vi "Adjust ROI.vi"(10 "Horizontal Pixel ROI IN":cluster{i64, i64}) -> (2 "Horizontal Pixel ROI OUT":cluster{i64, i64})   [LabVIEW 2020]
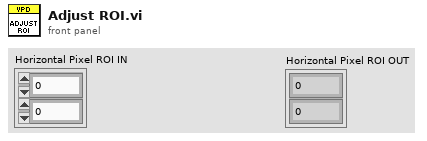
[diagram p1: front panel]
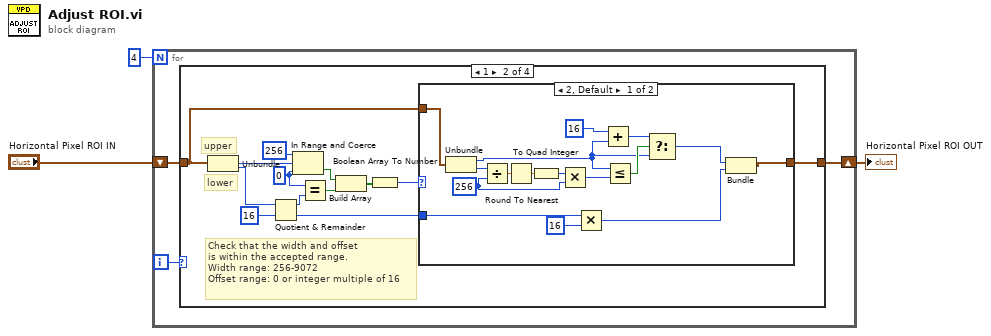
[diagram p0: block diagram]
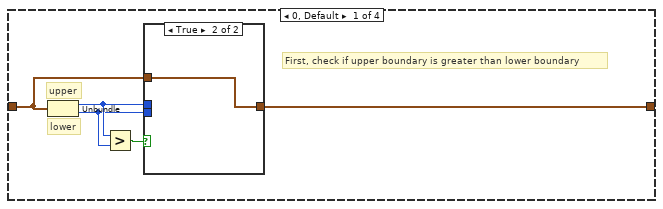
[diagram p2: hidden frame]
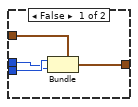
[diagram p3: hidden frame]
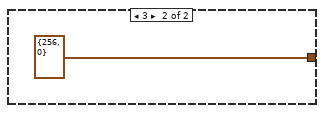
[diagram p4: hidden frame]
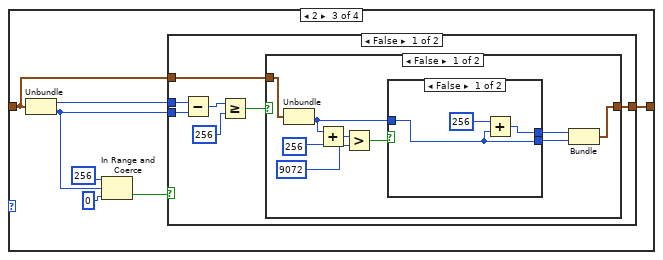
[diagram p5: hidden frame]
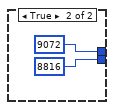
[diagram p6: hidden frame]
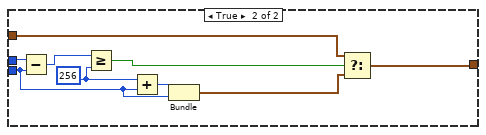
[diagram p8: hidden frame]
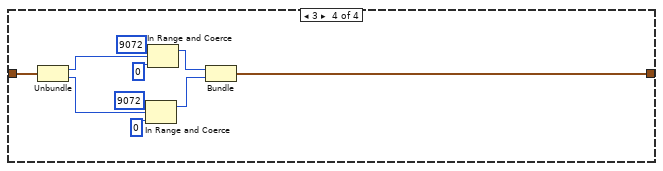
[diagram p9: hidden frame]
diagram:
  n1 = for {
    N: 4 -> [_]
    shift-right: [w5] -> w2
    shift-left: "Horizontal Pixel ROI IN" -> [w6]
    i -> [w4]
    n2 = case shown="1" w4 {
      tunnel: w6 -> [w10 w24 w48 w94]
      tunnel: [w7 w23 w47 w87] -> w5
      frame 0, Default {
        # "First, check if upper boundary is greater than lower boundary"
        # "lower"
        # "upper"
        n3 = Unbundle(w10) -> (w9:i64, w8:i64)
        n4 = Greater?(x=w9, y=w8) -> (0:w11:bool)
        n5 = case shown="True" w11 {
          tunnel: w10 -> [w15 w16]
          tunnel: w9 -> [w12 _]
          tunnel: w8 -> [w14 _]
          tunnel: [w13 w16] -> w7
          frame False {
            n6 = Bundle(cluster=w15, w14, w12) -> (w13:cluster{i64, i64})
          }
          frame True {
          }
        }
      }
      frame 1 {
        w19 = i64 0 ("lower limit")
        # "Check that the width and offset\nis within the accepted range.\nWidth range: 256-9072\nOffset range: 0 or integer multiple of 16"
        # "upper"
        # "lower"
        n7 = Unbundle(w24) -> (w29:i64, w22:i64)
        n8 = Quotient & Remainder(x=w22, y=i64 16) -> (x-y*floor(x/y)=w20:i64, floor(x/y)=w17:i64)
        n9 = In Range and Coerce(upper limit=i64 256, x=w29, lower limit=w19) -> (In Range?=w27:bool)  [unwired: 1 out]
        n10 = Equal?(x=w19, y=w20) -> (x = y?=w18:bool)
        n11 = Build Array(w27, w18) -> (w26:bool[])
        n12 = Boolean Array To Number(Boolean array=w26) -> (number=w25:u8)
        n13 = case shown="2, Default" w25 {
          tunnel: w24 -> [w33 _]
          tunnel: [w34 cluster{i64, i64} {256, 0} ("Horizontal Pixel slider")] -> w23
          tunnel: w17 -> [w32 _]
          frame 2, Default {
            w41 = i64 256 ("y")
            n14 = Unbundle(w33) -> (w38:i64, w45:i64)
            n15 = Divide(x=w45, y=w41) -> (x/y=w44:dbl)
            n16 = Round To Nearest(number=w44) -> (nearest integer value=w43:dbl)
            n17 = To Quad Integer(1:w43) -> (0:w42:i64)
            n18 = Multiply(x=w42, y=w41) -> (x*y=w36:i64)
            n19 = Multiply(x=w32, y=i64 16) -> (x*y=w30:i64)
            n20 = Add(x=i64 16, y=w38) -> (x+y=w39:i64)
            n21 = Less Or Equal?(x=w38, y=w36) -> (x <= y?=w40:bool)
            n22 = Select(t=w39, s=w40, f=w38) -> (s? t:f=w35:i64)
            n23 = Bundle(w35, w30) -> (w34:cluster{i64, i64})  [unwired: 1 in]
          }
          frame 3 {
          }
        }
      }
      frame 2 {
        n24 = Unbundle(w48) -> (w50:i64, w49:i64)
        n25 = In Range and Coerce(upper limit=i64 256, x=w49, lower limit=i64 0) -> (In Range?=w51:bool)  [unwired: 1 out]
        n26 = case shown="False" w51 {
          tunnel: w50 -> [w58 w84]
          tunnel: w49 -> [w59 w76]
          tunnel: w48 -> [w56 w81]
          tunnel: [w54 w80] -> w47
          frame False {
            n27 = Subtract(x=w58, y=w59) -> (x-y=w60:i64)
            n28 = Greater Or Equal?(x=w60, y=i64 256) -> (x >= y?=w55:bool)
            n29 = case shown="False" w55 {
              tunnel: w56 -> [w68 w75]
              tunnel: [w69 w75] -> w54
              frame False {
                n30 = Unbundle(w68) -> (w61:i64)  [unwired: 1 out]
                n31 = Add(x=w61, y=i64 256) -> (x+y=w66:i64)
                n32 = Greater?(x=w66, y=i64 9072) -> (0:w64:bool)
                n33 = case shown="False" w64 {
                  tunnel: [w72 i64 9072 ("y")] -> w63
                  tunnel: [w71 i64 8816 ("y")] -> w62
                  tunnel: w61 -> [w71 _]
                  frame False {
                    n34 = Add(x=i64 256, y=w71) -> (x+y=w72:i64)
                  }
                  frame True {
                  }
                }
                n35 = Bundle("y"=w63, "y"=w62) -> (w69:cluster{"y":i64, "y":i64})  [unwired: 1 in]
              }
              frame True {
              }
            }
          }
          frame True {
            w78 = i64 256 ("y")
            n36 = Subtract(x=w84, y=w76) -> (x-y=w83:i64)
            n37 = Greater Or Equal?(x=w83, y=w78) -> (x >= y?=w82:bool)
            n38 = Add(x=w78, y=w76) -> (x+y=w77:i64)
            n39 = Bundle(w77, w76) -> (w79:cluster{i64, i64})  [unwired: 1 in]
            n40 = Select(t=w81, s=w82, f=w79) -> (s? t:f=w80:cluster{i64, i64})
          }
        }
      }
      frame 3 {
        n41 = Unbundle(w94) -> (w88:i64, w91:i64)
        n42 = In Range and Coerce(upper limit=i64 9072, x=w91, lower limit=i64 0) -> (coerced(x)=w85:i64)  [unwired: 1 out]
        n43 = In Range and Coerce(upper limit=i64 9072, x=w88, lower limit=i64 0) -> (coerced(x)=w86:i64)  [unwired: 1 out]
        n44 = Bundle("upper limit"=w86, "upper limit"=w85) -> (w87:cluster{"upper limit":i64, "upper limit":i64})  [unwired: 1 in]
      }
    }
  }
  "Horizontal Pixel ROI OUT" <- w2
